vi "Close.vi"(8 "error in (no error)":errorcluster, 11 "VISA resource name":refnum<visa-resource-name>) -> (0 "error out":errorcluster)   [LabVIEW 2020, in "Agilent 33XXX Series.lvlib"]
doc: "Performs an instrument error query before terminating the software connection to the instrument."
uses:
  Agilent 33XXX Series.lvlib
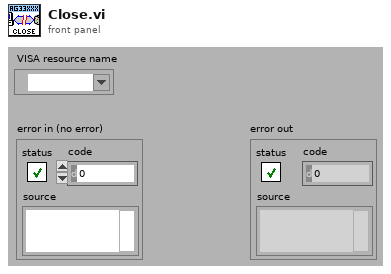
[diagram p1: front panel]
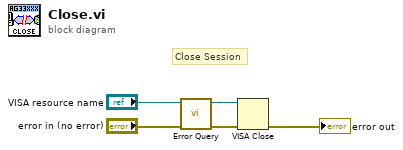
[diagram p0: block diagram]
diagram:
  # "Close Session"
  n1 = call "Error Query.vi"("error in (no error)"="error in (no error)", "VISA resource name"="VISA resource name") -> ("error out"=w5:errorcluster, "VISA resource name out"=w4:refnum<visa-resource-name>)  [unwired: 6 in, 2 out]
  n2 = VISA Close(VISA resource name=w4, error in (no error)=w5) -> (error out=→"error out":errorcluster)
